vi "XnPoints Concept - Digital Temp.vi"() -> ()   [LabVIEW 2014]
panel:
  in  "Automate":bool
  out "Thermometer_C":dbl(slide) scale=0.0..100.0
  out "Thermometer_B":dbl(slide) scale=0.0..100.0
  out "Thermometer_A":dbl(slide) scale=0.0..100.0
  in  "Pulse Time":dbl=1.0
  in  "Temp_C":bool
  in  "Temp_B":bool
  out "3.3V":refnum<vi>[](array[refnum])
  out "GND":refnum<vi>[](array[refnum])
  out "SCL":refnum<vi>[](array[refnum])
  out "SDA":refnum<vi>[](array[refnum])
  in  "Master":bool
  out "SCL_6":u32(colorbox)=16860
  out "SCL_7":u32(colorbox)=16860
  out "SCL_5":u32(colorbox)=16860
  out "SDA_7":u32(colorbox)=357120
  out "SDA_5":u32(colorbox)=357120
  out "SDA_6":u32(colorbox)=357120
  out "GND_6":u32(colorbox)=16777222
  out "GND_7":u32(colorbox)=16777222
  out "GND_5":u32(colorbox)=16777222
  out "3.3V_5":u32(colorbox)=16711680
  out "3.3V_7":u32(colorbox)=16711680
  out "3.3V_6":u32(colorbox)=16711680
  out "SCL_2":u32(colorbox)=16860
  out "SCL_4":u32(colorbox)=16860
  out "SCL_3":u32(colorbox)=16860
  out "SCL":u32(colorbox)=16860
  out "SDA_4":u32(colorbox)=357120
  out "SDA_3":u32(colorbox)=357120
  out "SDA_2":u32(colorbox)=357120
  out "SDA":u32(colorbox)=357120
  out "GND_4":u32(colorbox)
  out "GND_3":u32(colorbox)
  out "GND_2":u32(colorbox)
  out "GND":u32(colorbox)
  out "3.3V_4":u32(colorbox)=16711680
  out "3.3V_2":u32(colorbox)=16711680
  out "3.3V_3":u32(colorbox)=16711680
  out "3.3V":u32(colorbox)=16711680
  in  "temp":dbl=23.7
  in  "Message":enum16{"Status?", "Temp?", "Voltage?"}(ring)
  in  "Send":bool
  in  "Device Select":enum16{"Temp_A", "Temp_B", "Temp_C"}(ring)
  in  "Temp_A":bool
  in  "Stop Button":bool
  # "Digital Temperture Sensor"
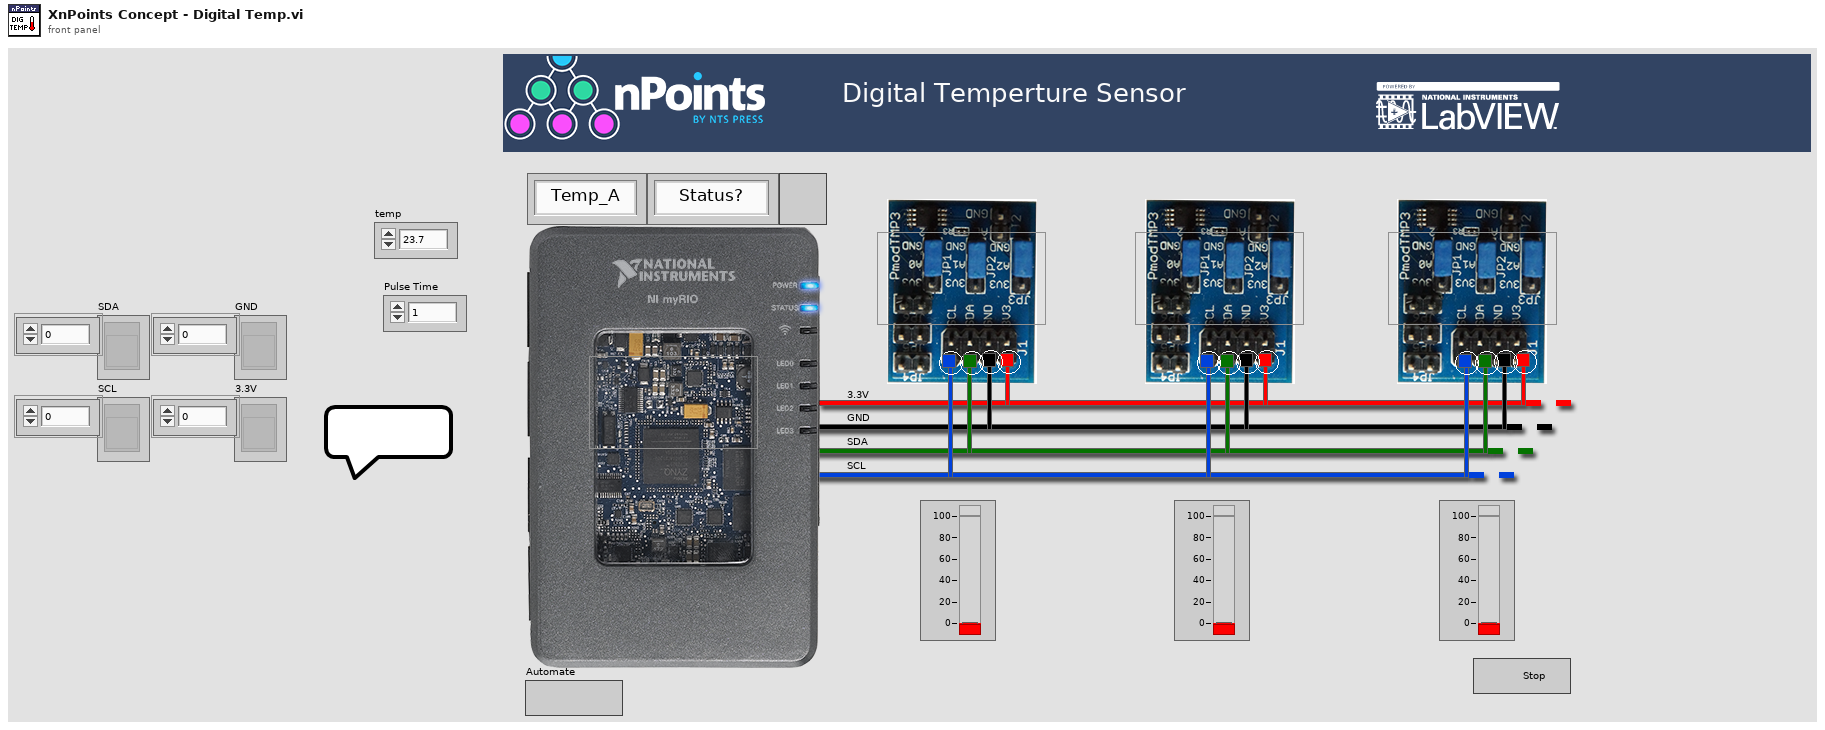
[diagram p1: front panel]
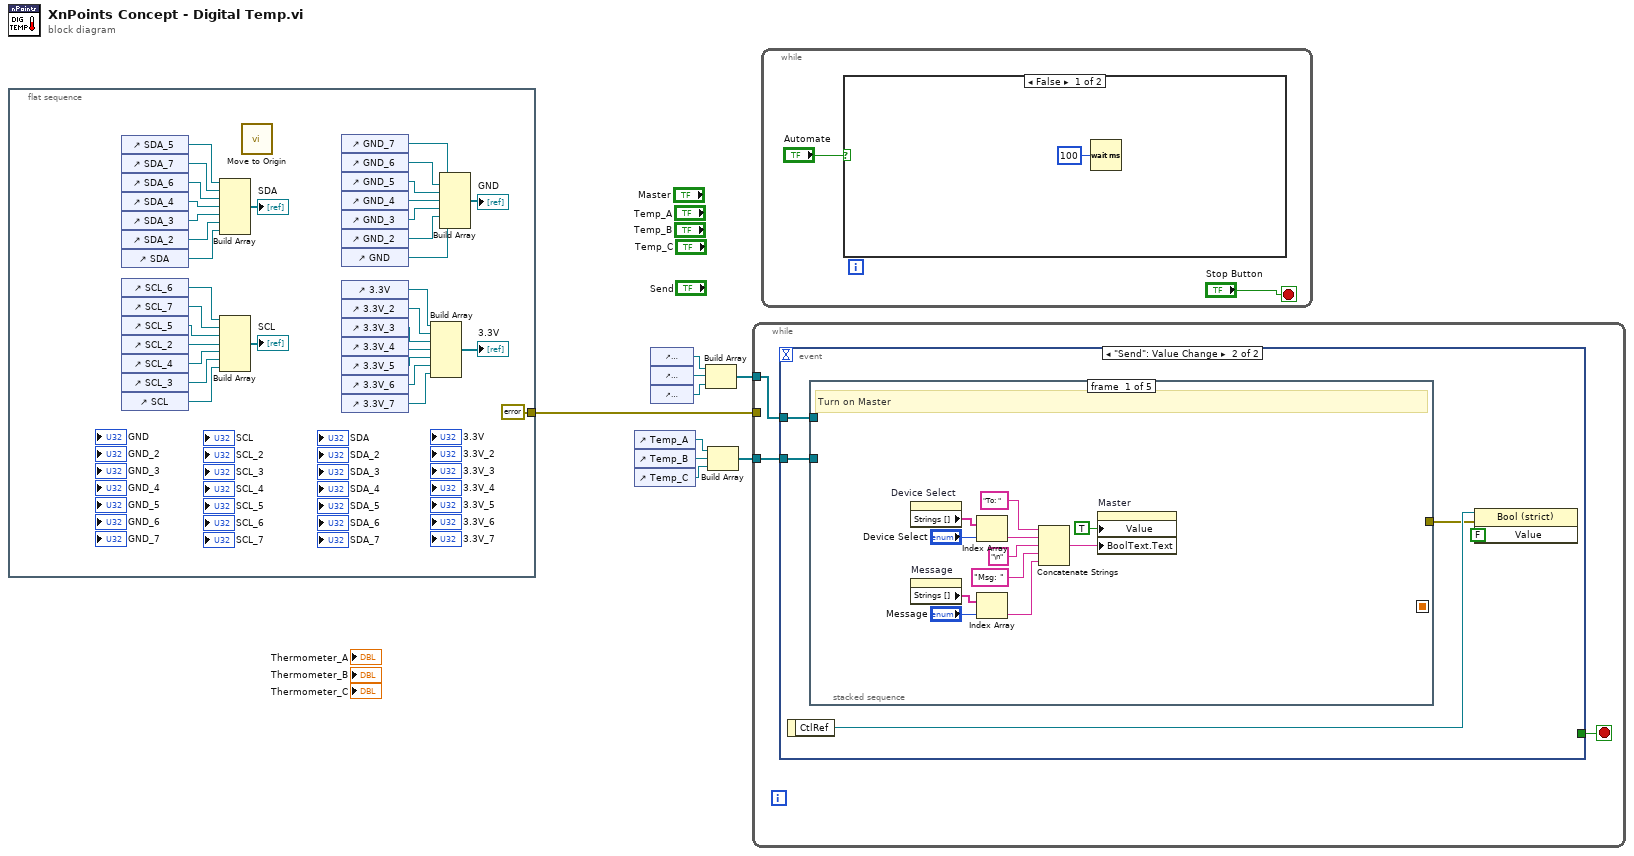
[diagram p0: block diagram]
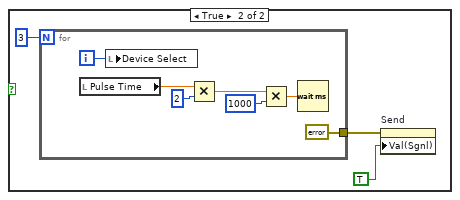
[diagram p2: hidden frame]
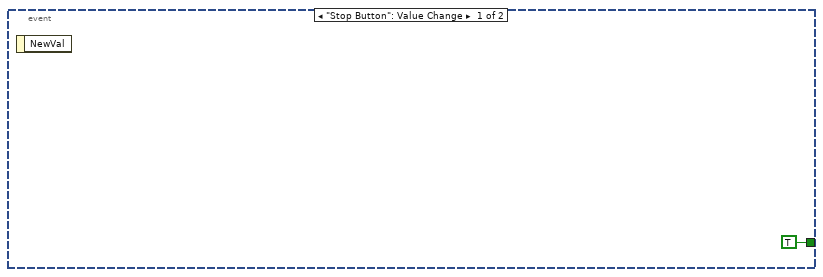
[diagram p3: hidden frame]
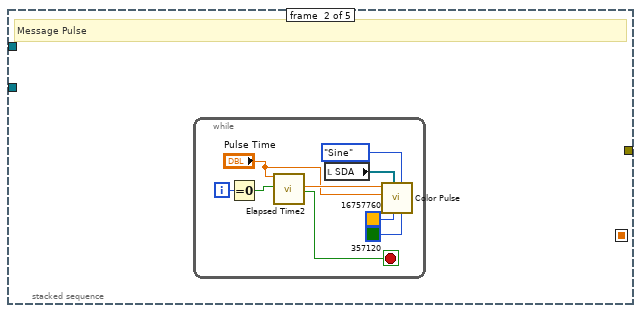
[diagram p4: hidden frame]
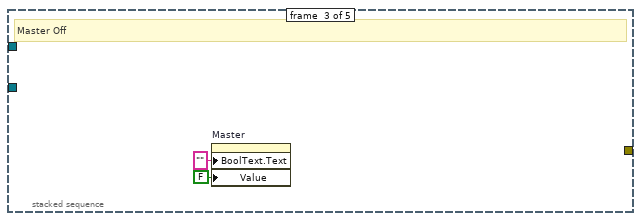
[diagram p5: hidden frame]
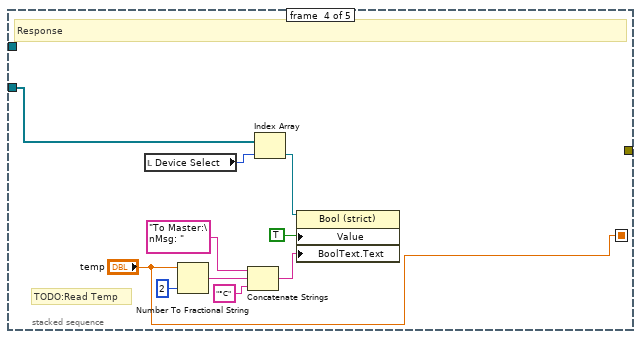
[diagram p6: hidden frame]
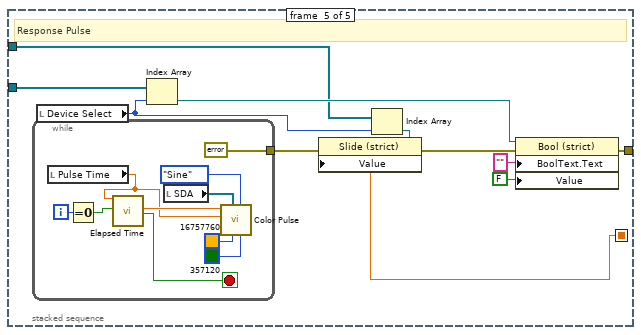
[diagram p7: hidden frame]
diagram:
  n1 = flat-sequence {
    tunnel: [errorcluster {"status"=FALSE, "code"=0, "source"=""} ("error constant")] -> w6
    frame #0 {
      n2 = control-ref of="SDA_5"() -> (w22:refnum<vi>)
      n3 = control-ref of="SDA_7"() -> (w23:refnum<vi>)
      n4 = control-ref of="SDA_6"() -> (w24:refnum<vi>)
      n5 = control-ref of="SDA_4"() -> (w28:refnum<vi>)
      n6 = control-ref of="SDA_3"() -> (w27:refnum<vi>)
      n7 = control-ref of="SDA_2"() -> (w26:refnum<vi>)
      n8 = control-ref of="SDA"() -> (w25:refnum<vi>)
      n9 = control-ref of="SCL_6"() -> (w35:refnum<vi>)
      n10 = control-ref of="SCL_7"() -> (w34:refnum<vi>)
      n11 = control-ref of="SCL_5"() -> (w33:refnum<vi>)
      n12 = control-ref of="SCL_2"() -> (w32:refnum<vi>)
      n13 = control-ref of="SCL_4"() -> (w31:refnum<vi>)
      n14 = control-ref of="SCL_3"() -> (w30:refnum<vi>)
      n15 = control-ref of="SCL"() -> (w29:refnum<vi>)
      n16 = Build Array(w22, w23, w24, w28, w27, w26, w25) -> (→"SDA":refnum<vi>[])
      n17 = Build Array(w35, w34, w33, w32, w31, w30, w29) -> (→"SCL":refnum<vi>[])
      n18 = call "Move to Origin.vi"() -> ()  [unwired: 3 in, 1 out]
      n19 = control-ref of="GND_7"() -> (w42:refnum<vi>)
      n20 = control-ref of="GND_6"() -> (w41:refnum<vi>)
      n21 = control-ref of="GND_5"() -> (w40:refnum<vi>)
      n22 = control-ref of="GND_4"() -> (w39:refnum<vi>)
      n23 = control-ref of="GND_3"() -> (w38:refnum<vi>)
      n24 = control-ref of="GND_2"() -> (w37:refnum<vi>)
      n25 = control-ref of="GND"() -> (w36:refnum<vi>)
      n26 = control-ref of="3.3V"() -> (w20:refnum<vi>)
      n27 = control-ref of="3.3V_2"() -> (w19:refnum<vi>)
      n28 = control-ref of="3.3V_3"() -> (w18:refnum<vi>)
      n29 = control-ref of="3.3V_4"() -> (w17:refnum<vi>)
      n30 = control-ref of="3.3V_5"() -> (w16:refnum<vi>)
      n31 = control-ref of="3.3V_6"() -> (w15:refnum<vi>)
      n32 = control-ref of="3.3V_7"() -> (w14:refnum<vi>)
      n33 = Build Array(w20, w19, w18, w17, w16, w15, w14) -> (→"3.3V":refnum<vi>[])
      n34 = Build Array(w42, w41, w40, w39, w38, w37, w36) -> (→"GND":refnum<vi>[])
    }
  }
  n35 = control-ref of="Temp_A"() -> (w7:refnum<vi>)
  n36 = control-ref of="Temp_B"() -> (w8:refnum<vi>)
  n37 = control-ref of="Temp_C"() -> (w9:refnum<vi>)
  n38 = control-ref of="Thermometer_A"() -> (w4:refnum<vi>)
  n39 = control-ref of="Thermometer_C"() -> (w3:refnum<vi>)
  n40 = control-ref of="Thermometer_B"() -> (w2:refnum<vi>)
  n41 = Build Array(w4, w3, w2) -> (w1:refnum<vi>[])
  n42 = Build Array(w7, w8, w9) -> (w5:refnum<vi>[])
  n43 = while {
    tunnel: w6 -> [_]
    tunnel: w5 -> [w44]
    tunnel: w1 -> [w43]
    stop <- w45 stop-if-true
    n44 = event shown="[1] \"Send\": Value Change" {
      selector: _ -> [_ _]
      dyn-events: _ -> [_ _]
      timeout: _ -> [_ _]
      tunnel: [TRUE _] -> w45
      tunnel: w44 -> [_ w51]
      tunnel: w43 -> [_ w47]
      event "Stop Button": Value Change {
        n45 = event-data() -> ()  [unwired: 1 in, 1 out]
      }
      event "Send": Value Change {
        n46 = event-data() -> ("CtlRef"=w50:refnum<vi>)  [unwired: 1 in]
        n47 = stacked-sequence {
          seq-local: [_ _ _ "temp" _] -> [_ _ _ _ w86]
          tunnel: w51 -> [_ _ _ w76 w92]
          tunnel: [_ _ _ _ w90] -> w48
          tunnel: w47 -> [_ _ _ _ w88]
          frame #0 {
            # "Turn on Master"
            n48 = property on="Device Select" class="Enum (strict)"() -> ("Strings []"=w54:string[])  [unwired: 2 in, 2 out]
            n49 = property on="Message" class="Enum (strict)"() -> ("Strings []"=w53:string[])  [unwired: 2 in, 2 out]
            n50 = Index Array(array=w54, index="Device Select") -> (element=w58:string)
            n51 = Index Array(array=w53, index="Message") -> (element=w61:string)
            n52 = Concatenate Strings("To: " ("Boolean Text.Text"), w58, "\n" ("string"), "Msg: " ("Boolean Text.Text"), w61) -> (w56:string)
            n53 = property on="Master" class="Bool (strict)"("Value"=TRUE ("Master"), "BoolText.Text"=w56) -> ()  [unwired: 2 in, 2 out]
          }
          frame #1 {
            # "Message Pulse"
            n54 = while {
              i -> [w65]
              stop <- w68 stop-if-true
              n55 = Equal To 0?(x=w65) -> (x = 0?=w64:bool)
              n56 = call "Elapsed Time2"("Time Target (s)"="Pulse Time", "Reset"=w64) -> ("Elapsed Time (s)"=w69:dbl, "Time has Elapsed"=w68:bool)  [unwired: 10 in, 6 out]
              n57 = local read "SDA"() -> (w71:refnum<vi>[])
              n58 = call "Color Pulse.vi"("Color 2"=u32 357120, "Style"=enum16{"Sine", "Square", "Sawtooth", "Triangle"}."Sine", "Color 1"=u32 16757760, "Array"=w71, "Pulse Period"="Pulse Time", "Elapsed Time (s)"=w69) -> ()  [unwired: 5 in, 1 out]
            }
          }
          frame #2 {
            # "Master Off"
            n59 = property on="Master" class="Bool (strict)"("BoolText.Text"="" ("Boolean Text.Text"), "Value"=FALSE ("Master")) -> ()  [unwired: 2 in, 2 out]
          }
          frame #3 {
            # "TODO:Read Temp"
            # "Response"
            n60 = local read "Device Select"() -> (w77:enum16{"Temp_A", "Temp_B", "Temp_C"})
            n61 = Number To Fractional String(number="temp", precision (6)=i16 2) -> (F-format string=w80:string)  [unwired: 2 in]
            n62 = Concatenate Strings("To Master:\nMsg: " ("Boolean Text.Text"), w80, "°C" ("Boolean Text.Text")) -> (w78:string)
            n63 = Index Array(array=w76, index=w77) -> (element=w75:refnum<vi>)
            n64 = property on="Property Node" class="Bool (strict)"(reference=w75, "Value"=TRUE ("Master"), "BoolText.Text"=w78) -> ()  [unwired: 1 in, 2 out]
          }
          frame #4 {
            # "Response Pulse"
            n65 = while {
              tunnel: [errorcluster {"status"=FALSE, "code"=0, "source"=""} ("error in (no error)")] -> w85
              i -> [w98]
              stop <- w101 stop-if-true
              n66 = local read "Pulse Time"() -> (w96:dbl)
              n67 = Equal To 0?(x=w98) -> (x = 0?=w97:bool)
              n68 = call "Elapsed Time"("Time Target (s)"=w96, "Reset"=w97) -> ("Elapsed Time (s)"=w102:dbl, "Time has Elapsed"=w101:bool)  [unwired: 10 in, 6 out]
              n69 = local read "SDA"() -> (w104:refnum<vi>[])
              n70 = call "Color Pulse.vi"("Color 2"=u32 357120, "Style"=enum16{"Sine", "Square", "Sawtooth", "Triangle"}."Sine", "Color 1"=u32 16757760, "Array"=w104, "Pulse Period"=w96, "Elapsed Time (s)"=w102) -> ()  [unwired: 5 in, 1 out]
            }
            n71 = local read "Device Select"() -> (w89:enum16{"Temp_A", "Temp_B", "Temp_C"})
            n72 = Index Array(array=w92, index=w89) -> (element=w91:refnum<vi>)
            n73 = Index Array(array=w88, index=w89) -> (element=w87:refnum<vi>)
            n74 = property on="Property Node" class="Slide (strict)"(reference=w87, error in=w85, "Value"=w86) -> (error out=w84:errorcluster)  [unwired: 1 out]
            n75 = property on="Property Node" class="Bool (strict)"(reference=w91, error in=w84, "BoolText.Text"="" ("Boolean Text.Text"), "Value"=FALSE ("Master")) -> (error out=w90:errorcluster)  [unwired: 1 out]
          }
        }
        n76 = property on="Property Node" class="Bool (strict)"(reference=w50, error in=w48, "Value"=FALSE ("Master")) -> ()  [unwired: 2 out]
      }
    }
  }
  n77 = while {
    stop <- "Stop Button" stop-if-true
    n78 = case shown="False" "Automate" {
      frame False {
        n79 = Wait (ms)(milliseconds to wait=u32 100) -> ()  [unwired: 1 out]
      }
      frame True {
        n80 = for {
          N: 3 -> [_]
          tunnel: [errorcluster {"status"=FALSE, "code"=0, "source"=""} ("error in (no error)")] -> w109
          i -> [w117]
          n81 = local read "Pulse Time"() -> (w113:dbl)
          n82 = local write "Device Select"(w117) -> ()
          n83 = Multiply(x=w113, y=2) -> (x*y=w114:dbl)
          n84 = Multiply(x=w114, y=1000) -> (x*y=w115:dbl)
          n85 = Wait (ms)(milliseconds to wait=w115) -> ()  [unwired: 1 out]
        }
        n86 = property on="Send" class="Bool (strict)"(error in=w109, "Val(Sgnl)"=TRUE ("Value (Signaling)")) -> ()  [unwired: 1 in, 2 out]
      }
    }
  }
